vi "Untitled 8.vi"() -> ()   [LabVIEW 2023]
panel:
  out "Time":u32
  in  "Reset/Count":bool=TRUE
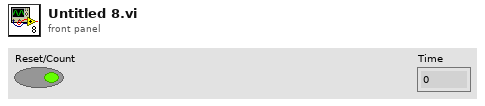
[diagram p1: front panel]
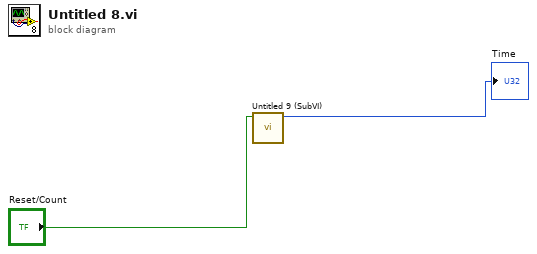
[diagram p0: block diagram]
diagram:
  n1 = call "Untitled 9 (SubVI).vi"("Reset/Count"="Reset/Count") -> ("Numeric"=→"Time":u32)  [unwired: 10 in]
